vi "SP Check Limit X, x0, dx.vi"(0 "X":dbl[](array[numeric]) format="%0.2f", 1 "x0":dbl format="%0.2f", 2 "dX":dbl format="%0.2f", 3 "error in":errorcluster, 4 "Check x0? (T)":bool=TRUE) -> (8 "Limit Spec OK":bool, 10 "error out":errorcluster)   [LabVIEW 2011]
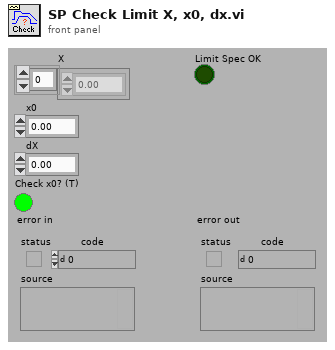
[diagram p1: front panel]
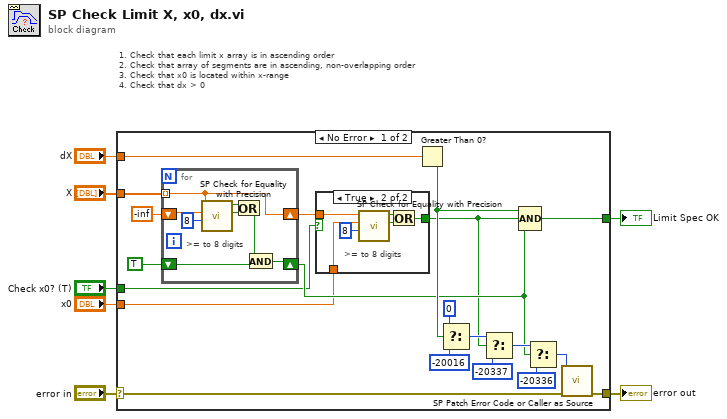
[diagram p0: block diagram]
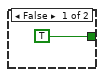
[diagram p2: hidden frame]
diagram:
  # "1. Check that each limit x array is in ascending order\n2. Check that array of segments are in ascending, non-overlapping order\n3. Check that x0 is located within x-range\n4. Check that dx > 0"
  n1 = case shown="No Error" "error in" {
    selector: "error in" -> [w14 w43]
    tunnel: [w25 w43] -> w6
    tunnel: [w13 _] -> w5
    tunnel: "X" -> [w12 _]
    tunnel: "dX" -> [w11 _]
    tunnel: "x0" -> [w10 _]
    tunnel: "Check x0? (T)" -> [w8 _]
    frame No Error {
      n2 = for {
        shift-right: [w36] -> w16
        shift-left: -inf -> [w41]
        tunnel: w12 -> [w36] mode=indexing
        shift-right: [w35] -> w15
        shift-left: TRUE -> [w42]
        # ">= to 8 digits"
        n3 = call "SP Check for Equality with Precision.vi"("precision"=8, "n2"=w41, "n1"=w36) -> ("n1 > n2?"=w39:bool, "equal (within precision)"=w40:bool)  [unwired: 7 out]
        n4 = Or(x=w40, y=w39) -> (x .or. y?=w38:bool)
        n5 = And(x=w38, y=w42) -> (x .and. y?=w35:bool)
      }
      n6 = case shown="True" w8 {
        tunnel: w16 -> [_ w33]
        tunnel: w10 -> [_ w30]
        tunnel: [TRUE ("x .or. y?") w29] -> w9
        frame False {
        }
        frame True {
          # ">= to 8 digits"
          n7 = call "SP Check for Equality with Precision.vi"("precision"=8, "n2"=w30, "n1"=w33) -> ("n1 > n2?"=w31:bool, "equal (within precision)"=w32:bool)  [unwired: 7 out]
          n8 = Or(x=w32, y=w31) -> (x .or. y?=w29:bool)
        }
      }
      n9 = Greater Than 0?(x=w11) -> (x > 0?=w18:bool)
      n10 = Select(t=0 ("Error Code"), s=w18, f=-20016) -> (s? t:f=w19:i32)
      n11 = Select(t=w19, s=w9, f=-20337 ("Error Code")) -> (s? t:f=w23:i32)
      n12 = Compound Arithmetic op=AND(w18, w9, w15) -> (w13:bool)
      n13 = Select(t=w23, s=w15, f=-20336 ("Error Code")) -> (s? t:f=w17:i32)
      n14 = call "SP Patch Error Code or Caller as Source.vi"("error in (no error)"=w14, "error code"=w17) -> ("error out"=w25:errorcluster)  [unwired: 2 in, 7 out]
    }
    frame Error {
    }
  }
  "error out" <- w6
  "Limit Spec OK" <- w5
